vi "Writing by index.vi"(5 "refnum in":refnum<file>, 6 "error in":errorcluster, 8 "Input array":sgl[][](array[numeric]), 9 "While Equal to index":sgl) -> (0 "error out":errorcluster, 3 "Subarray Size":i32, 4 "refnum out":refnum<file>)   [LabVIEW 2020]
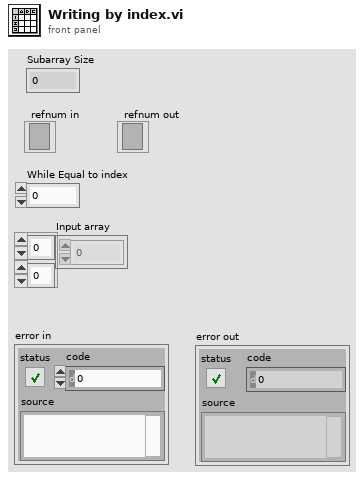
[diagram p1: front panel]
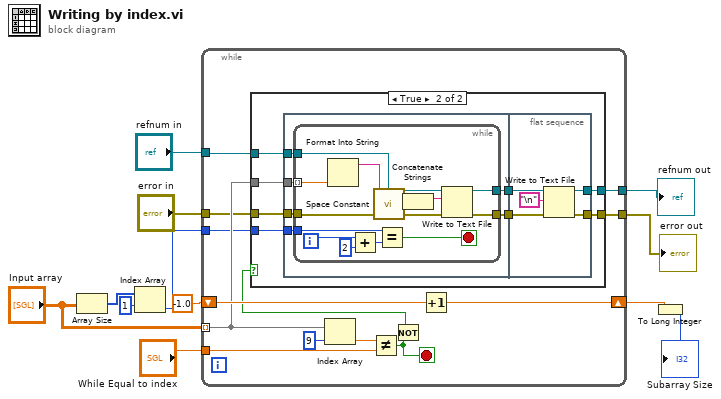
[diagram p0: block diagram]
diagram:
  n1 = Array Size(array="Input array") -> (size(s)=w3:i32[])
  n2 = Index Array(array=w3, index=1) -> (element=w1:i32)
  n3 = while {
    tunnel: "Input array" -> [w21] mode=indexing
    shift-right: [w22] -> w10
    shift-left: -1.0 -> [w23]
    tunnel: "While Equal to index" -> [w20]
    tunnel: "refnum in" -> [w19]
    tunnel: [w18] -> w7
    tunnel: [w17] -> w5
    tunnel: "error in" -> [w16]
    tunnel: w1 -> [w15]
    stop <- w14 stop-if-true
    n4 = Index Array(array=w21, index=9) -> (element=w25:sgl)
    n5 = Not Equal?(x=w25, y=w20) -> (x != y?=w14:bool)
    n6 = Not(x=w14) -> (.not. x?=w13:bool)
    n7 = case shown="True" w13 {
      tunnel: w21 -> [_ w33]
      tunnel: w19 -> [w27 w32]
      tunnel: [w27 w31] -> w18
      tunnel: [w26 w30] -> w17
      tunnel: w16 -> [w26 w29]
      tunnel: w15 -> [_ w28]
      frame False {
      }
      frame True {
        n8 = flat-sequence {
          tunnel: w33 -> [w41]
          tunnel: w32 -> [w40]
          tunnel: w29 -> [w37]
          tunnel: w28 -> [w36]
          tunnel: [w39] -> w35
          tunnel: [w38] -> w34
          tunnel: [w58] -> w30
          tunnel: [w59] -> w31
          tunnel: w35 -> [w56]
          tunnel: w34 -> [w57]
          frame #0 {
            n9 = while {
              tunnel: w41 -> [w47] mode=indexing
              tunnel: w40 -> [w51]
              tunnel: [w50] -> w39
              tunnel: [w49] -> w38
              tunnel: w37 -> [w48]
              tunnel: w36 -> [w46]
              i -> [w42]
              stop <- w45 stop-if-true
              n10 = Format Into String(w47) -> (resulting string=w52:string)  [unwired: 3 in, 1 out]
              n11 = Add(x=w42, y=2) -> (x+y=w43:i32)
              n12 = call <vilib>:"Space Constant.vi"() -> ("String"=w54:string)
              n13 = Equal?(x=w46, y=w43) -> (x = y?=w45:bool)
              n14 = Concatenate Strings(w52, w54) -> (w53:string)
              n15 = Write to Text File(file (use dialog)=w51, text=w53, error in=w48) -> (refnum out=w50:refnum<file>, error out=w49:errorcluster)  [unwired: 1 in, 1 out]
            }
          }
          frame #1 {
            n16 = Write to Text File(file (use dialog)=w56, text="\n", error in=w57) -> (refnum out=w59:refnum<file>, error out=w58:errorcluster)  [unwired: 1 in, 1 out]
          }
        }
      }
    }
    n17 = Increment(x=w23) -> (x+1=w22:dbl)
  }
  "refnum out" <- w7
  "error out" <- w5
  n18 = To Long Integer(number=w10) -> (32bit integer=→"Subarray Size":i32)
